vi "mian .vi"() -> ()   [LabVIEW 2013]
panel:
  out "机器ID":string="F3XS67WZ8BAQ"
  in  "密钥":u32=1308622971
  in  "VD":T1
  in  "PLC 系列":u8(ring) items=["1200.200.200SMART"=0, "S7-300"=2, "S7-400"=3]
  in  "PLC IP":string="192.168.3.200"
  in  "VW":T2={"VW0"=30, "VW2"=0, "VW4"=0, "VW6"=0, "VW8"=0, "VW10"=0, "VW12"=0, "VW14"=0, "VW16"=0, "VW18"=0, "VW20"=0, "VW22"=0, "VW24"=0, "VW26"=0, "VW28"=0, "VW30"=0, "VW32"=0, "VW34"=0, "VW36"=0, "VW38"=0, "VW40"=0, "VW42"=0, "VW44"=0, "VW46"=0}
  out "RMD":T3
  in  "WMD":T4
  out "RQD":T3={"Y20 2"=FALSE, "Y21 2"=FALSE, "Y22 2"=FALSE, "Y24 2"=FALSE, "Y23 2"=FALSE, "Y25 2"=FALSE, "Y26 2"=FALSE, "Y27 2"=FALSE, "Y10 2"=FALSE, "Y11 2"=FALSE, "Y12 2"=FALSE, "Y13 2"=FALSE, "Y14 2"=FALSE, "Y15 2"=FALSE, "Y16 2"=FALSE, "Y17 2"=FALSE, "Y0 2"=TRUE, "Y1 2"=TRUE, "Y2 2"=TRUE, "Y3 2"=TRUE, "Y4 2"=TRUE, "Y5 2"=FALSE, "Y6 2"=FALSE, "Y7 2"=FALSE, "Y30 2"=FALSE, "Y31 2"=FALSE, "Y32 2"=FALSE, "Y33 2"=FALSE, "Y34  2"=FALSE, "Y35  2"=FALSE, "Y36 2"=FALSE, "Y37 2"=FALSE}
  in  "WQD":T4
  out "RID":T5
  in  "停止":bool
  # "MX.0"
  # "QX.0-QX.7"
  # "IX.0-IX.7"
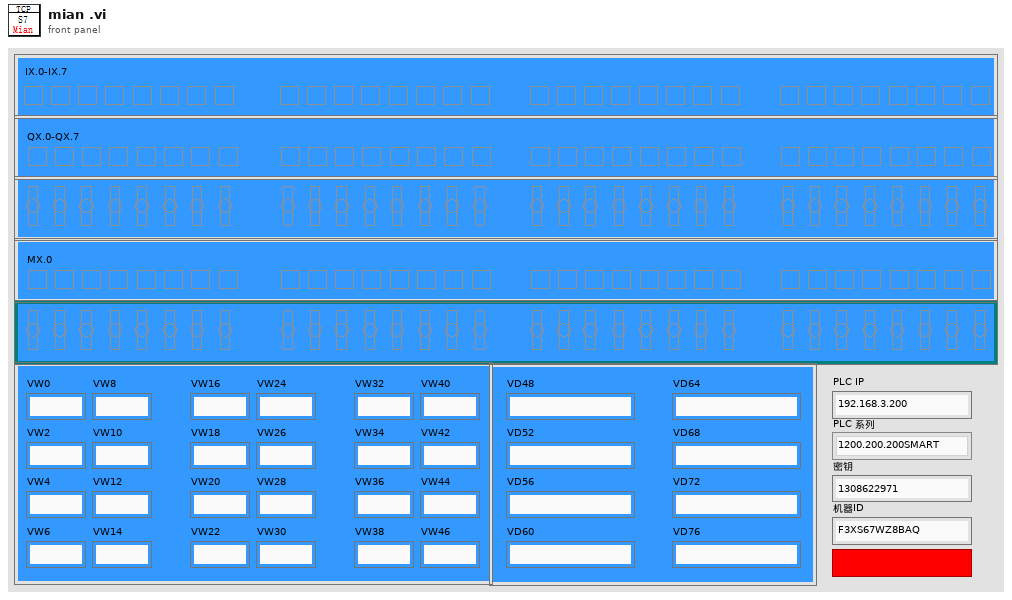
[diagram p1: front panel]
types:
  T1 = cluster{"VD48":u32, "VD52":u32, "VD56":u32, "VD60":u32, "VD64":u32, "VD68":u32, "VD72":u32, "VD76":u32}
  T2 = cluster{"VW0":u16, "VW2":u16, "VW4":u16, "VW6":u16, "VW8":u16, "VW10":u16, "VW12":u16, "VW14":u16, "VW16":u16, "VW18":u16, "VW20":u16, "VW22":u16, "VW24":u16, "VW26":u16, "VW28":u16, "VW30":u16, "VW32":u16, "VW34":u16, "VW36":u16, "VW38":u16, "VW40":u16, "VW42":u16, "VW44":u16, "VW46":u16}
  T3 = cluster{"Y20 2":bool, "Y21 2":bool, "Y22 2":bool, "Y24 2":bool, "Y23 2":bool, "Y25 2":bool, "Y26 2":bool, "Y27 2":bool, "Y10 2":bool, "Y11 2":bool, "Y12 2":bool, "Y13 2":bool, "Y14 2":bool, "Y15 2":bool, "Y16 2":bool, "Y17 2":bool, "Y0 2":bool, "Y1 2":bool, "Y2 2":bool, "Y3 2":bool, "Y4 2":bool, "Y5 2":bool, "Y6 2":bool, "Y7 2":bool, "Y30 2":bool, "Y31 2":bool, "Y32 2":bool, "Y33 2":bool, "Y34  2":bool, "Y35  2":bool, "Y36 2":bool, "Y37 2":bool}
  T4 = cluster{"Q3.0":bool, "Q3.1":bool, "Q3.2":bool, "Q3.3":bool, "Q3.4":bool, "Q3.5":bool, "Q3.6":bool, "Q3.7":bool, "Q2.0":bool, "Q2.1":bool, "Q2.2":bool, "Q2.3":bool, "Q2.4":bool, "Q2.5":bool, "Q2.6":bool, "Q2.7":bool, "Q1.0":bool, "Q1.1":bool, "Q1.2":bool, "Q1.3":bool, "Q1.4":bool, "Q1.5":bool, "Q1.6":bool, "Q1.7":bool, "Q0.0":bool, "Q0.1":bool, "Q0.2":bool, "Q0.3":bool, "Q0.4":bool, "Q0.5":bool, "Q0.6":bool, "Q0.7":bool}
  T5 = cluster{"X20":bool, "X21":bool, "X22":bool, "X24":bool, "X23":bool, "X25":bool, "X26":bool, "X27":bool, "X10":bool, "X11":bool, "X12":bool, "X13":bool, "X14":bool, "X15":bool, "X16":bool, " X17":bool, "X0":bool, "X1":bool, "X2":bool, "X3":bool, "X4":bool, "X5":bool, "X6":bool, "X7":bool, "X30":bool, "X31":bool, "X32":bool, "X33":bool, "X34 ":bool, "X35 ":bool, "X36":bool, "X37":bool}
  T6 = typedef "运行步骤控件.ctl" = enum16{"RI", "RQ", "RM", "RV"}
  T7 = cluster{"Boolean array[0]":bool, "Boolean array[1]":bool, "Boolean array[2]":bool, "Boolean array[3]":bool, "Boolean array[4]":bool, "Boolean array[5]":bool, "Boolean array[6]":bool, "Boolean array[7]":bool, "Boolean array[8]":bool, "Boolean array[9]":bool, "Boolean array[10]":bool, "Boolean array[11]":bool, "Boolean array[12]":bool, "Boolean array[13]":bool, "Boolean array[14]":bool, "Boolean array[15]":bool, "Boolean array[16]":bool, "Boolean array[17]":bool, "Boolean array[18]":bool, "Boolean array[19]":bool, "Boolean array[20]":bool, "Boolean array[21]":bool, "Boolean array[22]":bool, "Boolean array[23]":bool, "Boolean array[24]":bool, "Boolean array[25]":bool, "Boolean array[26]":bool, "Boolean array[27]":bool, "Boolean array[28]":bool, "Boolean array[29]":bool, "Boolean array[30]":bool, "Boolean array[31]":bool}
  T8 = cluster{"[0]":u32, "[1]":u32, "[2]":u32, "[3]":u32, "[4]":u32, "[5]":u32, "[6]":u32, "[7]":u32}
  T9 = cluster{"[0]":u16, "[1]":u16, "[2]":u16, "[3]":u16, "[4]":u16, "[5]":u16, "[6]":u16, "[7]":u16, "[8]":u16, "[9]":u16, "[10]":u16, "[11]":u16, "[12]":u16, "[13]":u16, "[14]":u16, "[15]":u16, "[16]":u16, "[17]":u16, "[18]":u16, "[19]":u16, "[20]":u16, "[21]":u16, "[22]":u16, "[23]":u16}
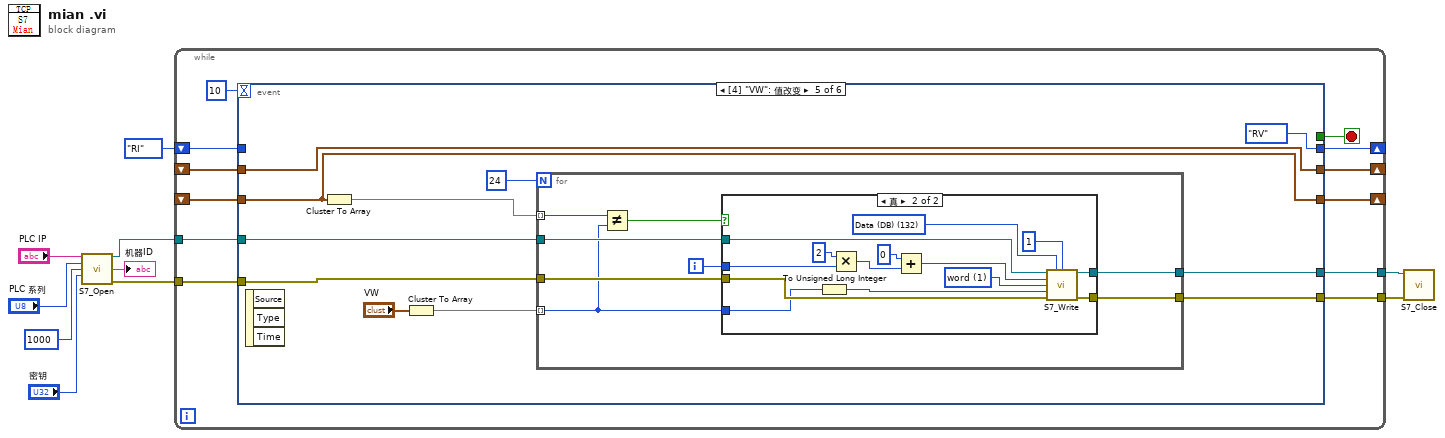
[diagram p0: block diagram]
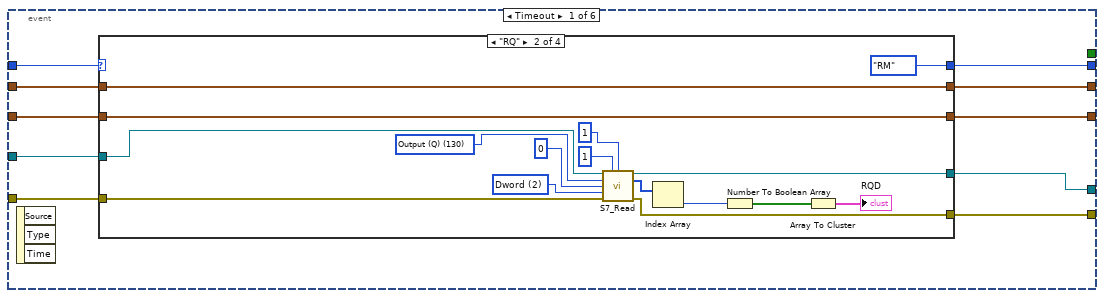
[diagram p2: hidden frame]
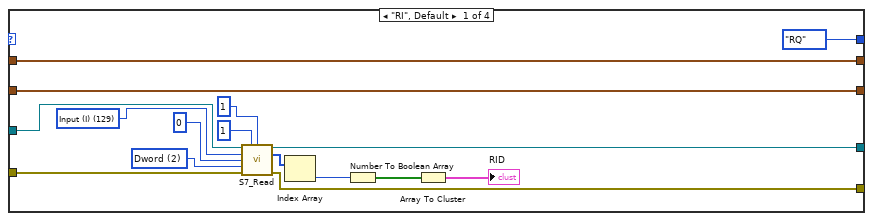
[diagram p3: hidden frame]
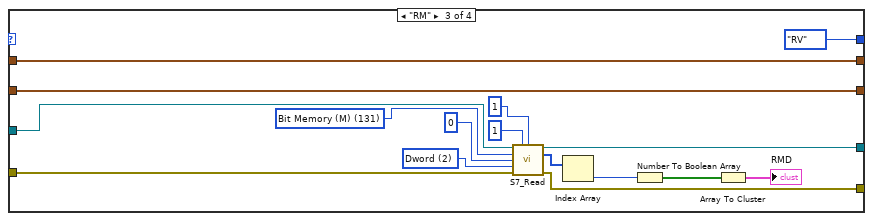
[diagram p4: hidden frame]
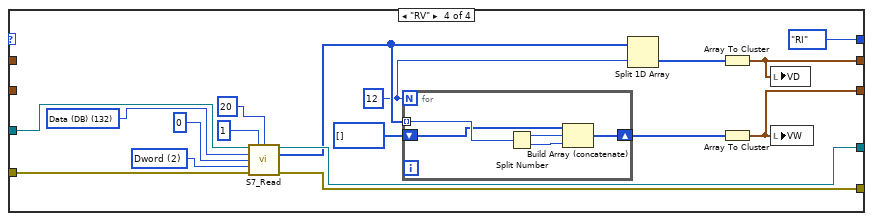
[diagram p5: hidden frame]
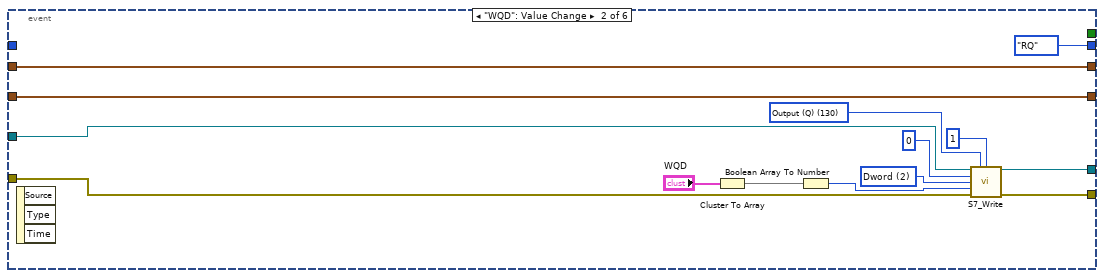
[diagram p6: hidden frame]
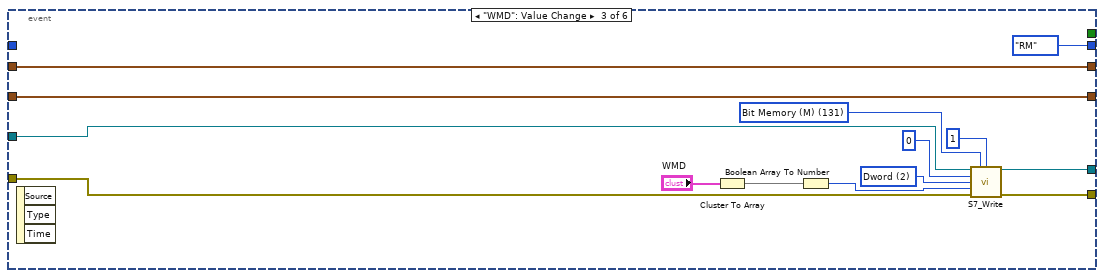
[diagram p7: hidden frame]
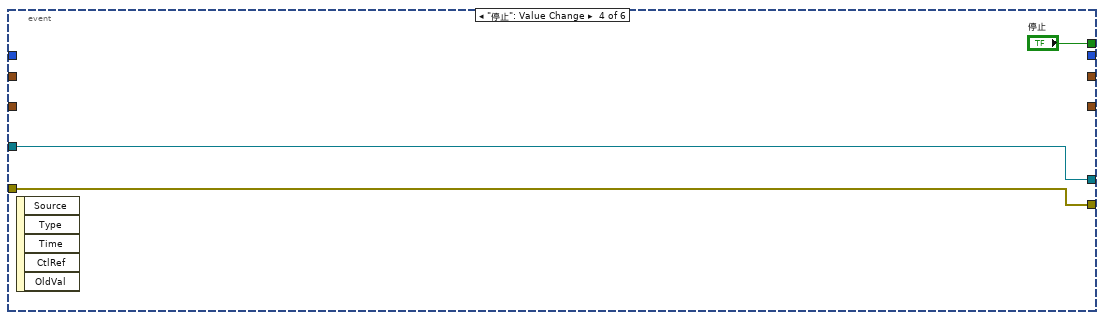
[diagram p8: hidden frame]
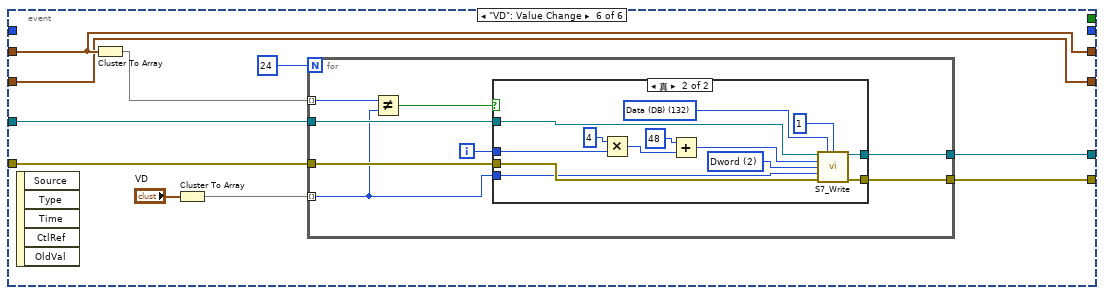
[diagram p10: hidden frame]
diagram:
  n1 = call "S7_Open.vi"("IP 地址"="PLC IP", "PLC 系列"="PLC 系列", "超时（MS）"=1000, "密钥"="密钥") -> ("TCP"=w9:refnum<k5>, "机器ID"=→"机器ID":string, "error out"=w8:errorcluster)  [unwired: 1 in, 8 out]
  n2 = while {
    tunnel: w9 -> [w21]
    tunnel: w8 -> [w20]
    tunnel: [w19] -> w7
    tunnel: [w18] -> w6
    shift-right: [w16] -> _
    shift-left: 运行步骤控件."RI" ("枚举") -> [w17]
    shift-right: [w15] -> _
    shift-left: _ -> [w13]
    shift-right: [w14] -> _
    shift-left: _ -> [w12]
    stop <- w11 stop-if-true
    n3 = event shown="[4] \"VW\": 值改变" {
      selector: _ -> [_ _ _ _ _ _]
      dyn-events: _ -> [_ _ _ _ _ _]
      timeout: 10 -> [_ _ _ _ _ _]
      tunnel: w21 -> [w32 w116 w122 w132 w142 w174]
      tunnel: w20 -> [w31 w115 w120 w131 w141 w173]
      tunnel: [w30 w114 w124 w132 w144 w172] -> w19
      tunnel: [w29 w113 w123 w131 w143 w171] -> w18
      tunnel: w17 -> [w28 _ _ _ _ _]
      tunnel: [w27 运行步骤控件."RQ" ("枚举") 运行步骤控件."RM" ("枚举") _ 运行步骤控件."RV" ("枚举") _] -> w16
      tunnel: [w26 w105 w119 _ w136 w169] -> w15
      tunnel: [w25 w104 w118 _ w135 w170] -> w14
      tunnel: w13 -> [w24 w105 w119 _ w136 w169]
      tunnel: w12 -> [w23 w104 w118 _ w135 w170]
      tunnel: [_ _ _ "停止" _ _] -> w11
      event Timeout {
        n4 = event-data() -> ()  [unwired: 4 out]
        n5 = case shown="\"RQ\"" w28 {
          tunnel: w32 -> [w44 w64 w72 w90]
          tunnel: w31 -> [w39 w63 w71 w89]
          tunnel: [w43 w62 w74 w92] -> w30
          tunnel: [w42 w61 w73 w91] -> w29
          tunnel: [运行步骤控件."RQ" ("枚举") 运行步骤控件."RM" ("枚举") 运行步骤控件."RV" ("枚举") 运行步骤控件."RI" ("枚举")] -> w27
          tunnel: [w34 w50 w66 w83] -> w26
          tunnel: [w33 w49 w65 w82] -> w25
          tunnel: w24 -> [w34 w50 w66 _]
          tunnel: w23 -> [w33 w49 w65 _]
          frame "RI", Default {
            w45 = u16 2 items=["byte", "word", "Dword"] ("数据类型")
            w41 = u8 129 items=["I/O (P)"=128, "Input (I)"=129, "Output (Q)"=130, "Bit Memory (M)"=131, "Data (DB)"=132, "Instance Data (DI)"=133, "Local Data (L)"=134, "Predecessor Local Data (VL)"=135] ("寄存器类型")
            n6 = call "S7_Read.vi"("TCP"=w44, "DB #"=u16 1, "读取长度"=u16 1, "寄存器类型"=w41, "起始地址"=u32 0, "数据类型"=w45, "error in"=w39) -> ("TCP"=w43:refnum<k5>, "数据"=w37:u32[], "error out"=w42:errorcluster)  [unwired: 6 out]
            n7 = Index Array(array=w37) -> (element=w36:u32)  [unwired: 1 in]
            n8 = Number To Boolean Array(number=w36) -> (Boolean array=w35:bool[])
            n9 = Array To Cluster(array=w35) -> (cluster=→"RID":T7)
          }
          frame "RQ" {
            w56 = u16 2 items=["byte", "word", "Dword"] ("数据类型")
            w58 = u8 130 items=["I/O (P)"=128, "Input (I)"=129, "Output (Q)"=130, "Bit Memory (M)"=131, "Data (DB)"=132, "Instance Data (DI)"=133, "Local Data (L)"=134, "Predecessor Local Data (VL)"=135] ("寄存器类型")
            n10 = call "S7_Read.vi"("TCP"=w64, "DB #"=u16 1, "读取长度"=u16 1, "寄存器类型"=w58, "起始地址"=u32 0, "数据类型"=w56, "error in"=w63) -> ("TCP"=w62:refnum<k5>, "数据"=w54:u32[], "error out"=w61:errorcluster)  [unwired: 6 out]
            n11 = Index Array(array=w54) -> (element=w53:u32)  [unwired: 1 in]
            n12 = Number To Boolean Array(number=w53) -> (Boolean array=w52:bool[])
            n13 = Array To Cluster(array=w52) -> (cluster=→"RQD":T7)
          }
          frame "RM" {
            w75 = u16 2 items=["byte", "word", "Dword"] ("数据类型")
            w79 = u8 131 items=["I/O (P)"=128, "Input (I)"=129, "Output (Q)"=130, "Bit Memory (M)"=131, "Data (DB)"=132, "Instance Data (DI)"=133, "Local Data (L)"=134, "Predecessor Local Data (VL)"=135] ("寄存器类型")
            n14 = call "S7_Read.vi"("TCP"=w72, "DB #"=u16 1, "读取长度"=u16 1, "寄存器类型"=w79, "起始地址"=u32 0, "数据类型"=w75, "error in"=w71) -> ("TCP"=w74:refnum<k5>, "数据"=w68:u32[], "error out"=w73:errorcluster)  [unwired: 6 out]
            n15 = Index Array(array=w68) -> (element=w70:u32)  [unwired: 1 in]
            n16 = Number To Boolean Array(number=w70) -> (Boolean array=w69:bool[])
            n17 = Array To Cluster(array=w69) -> (cluster=→"RMD":T7)
          }
          frame "RV" {
            w93 = u16 2 items=["byte", "word", "Dword"] ("数据类型")
            w97 = u8 132 items=["I/O (P)"=128, "Input (I)"=129, "Output (Q)"=130, "Bit Memory (M)"=131, "Data (DB)"=132, "Instance Data (DI)"=133, "Local Data (L)"=134, "Predecessor Local Data (VL)"=135] ("寄存器类型")
            w81 = 12
            n18 = call "S7_Read.vi"("TCP"=w90, "DB #"=u16 1, "读取长度"=u16 20, "寄存器类型"=w97, "起始地址"=u32 0, "数据类型"=w93, "error in"=w89) -> ("TCP"=w92:refnum<k5>, "数据"=w86:u32[], "error out"=w91:errorcluster)  [unwired: 6 out]
            n19 = for {
              N: w81 -> [_]
              tunnel: w86 -> [w102] mode=indexing
              shift-right: [w101] -> w85
              shift-left: u16[] [] -> [w100]
              n20 = Split Number(x=w102) -> (hi(x)=w99:u16, lo(x)=w98:u16)
              n21 = Build Array (concatenate)(w100, w99, w98) -> (w101:u16[])
            }
            n22 = Split 1D Array(array=w86, index=w81) -> (second subarray=w84:u32[])  [unwired: 1 out]
            n23 = Array To Cluster(array=w84) -> (cluster=w82:T8)
            n24 = Array To Cluster(array=w85) -> (cluster=w83:T9)
            n25 = local write "VD"(w82) -> ()
            n26 = local write "VW"(w83) -> ()
          }
        }
      }
      event "WQD": Value Change {
        w109 = u16 2 items=["byte", "word", "Dword"] ("数据类型")
        w112 = u8 130 items=["I/O (P)"=128, "Input (I)"=129, "Output (Q)"=130, "Bit Memory (M)"=131, "Data (DB)"=132, "Instance Data (DI)"=133, "Local Data (L)"=134, "Predecessor Local Data (VL)"=135] ("寄存器类型")
        n27 = event-data() -> ()  [unwired: 4 out]
        n28 = Cluster To Array(cluster="WQD") -> (array=w107:bool[])
        n29 = Boolean Array To Number(Boolean array=w107) -> (number=w106:u32)
        n30 = call "S7_Write.vi"("TCP"=w116, "寄存器类型"=w112, "DB #"=u16 1, "写入地址"=u32 0, "数据类型"=w109, "写入数据"=w106, "error in"=w115) -> ("TCP"=w114:refnum<k5>, "error out"=w113:errorcluster)  [unwired: 7 out]
      }
      event "WMD": Value Change {
        w127 = u16 2 items=["byte", "word", "Dword"] ("数据类型")
        w130 = u8 131 items=["I/O (P)"=128, "Input (I)"=129, "Output (Q)"=130, "Bit Memory (M)"=131, "Data (DB)"=132, "Instance Data (DI)"=133, "Local Data (L)"=134, "Predecessor Local Data (VL)"=135] ("寄存器类型")
        n31 = event-data() -> ()  [unwired: 4 out]
        n32 = Cluster To Array(cluster="WMD") -> (array=w126:bool[])
        n33 = Boolean Array To Number(Boolean array=w126) -> (number=w125:u32)
        n34 = call "S7_Write.vi"("TCP"=w122, "寄存器类型"=w130, "DB #"=u16 1, "写入地址"=u32 0, "数据类型"=w127, "写入数据"=w125, "error in"=w120) -> ("TCP"=w124:refnum<k5>, "error out"=w123:errorcluster)  [unwired: 7 out]
      }
      event "停止": Value Change {
        n35 = event-data() -> ()  [unwired: 6 out]
      }
      event "VW": Value Change {
        n36 = event-data() -> ()  [unwired: 4 out]
        n37 = Cluster To Array(cluster=w136) -> (array=w138:u16[])
        n38 = Cluster To Array(cluster="VW") -> (array=w137:u16[])
        n39 = for {
          N: 24 -> [_]
          tunnel: [w152] -> w144
          tunnel: [w151] -> w143
          tunnel: w142 -> [w150]
          tunnel: w141 -> [w149]
          tunnel: w138 -> [w148] mode=indexing
          tunnel: w137 -> [w146] mode=indexing
          i -> [w145]
          n40 = Not Equal?(x=w148, y=w146) -> (x != y?=w147:bool)
          n41 = case shown="真" w147 {
            tunnel: [w154 w165] -> w152
            tunnel: [w153 w164] -> w151
            tunnel: w150 -> [w154 w163]
            tunnel: w149 -> [w153 w162]
            tunnel: w146 -> [_ w157]
            tunnel: w145 -> [_ w159]
            frame False {
            }
            frame True {
              w166 = u16 1 items=["byte", "word", "Dword"] ("数据类型")
              w168 = u8 132 items=["I/O (P)"=128, "Input (I)"=129, "Output (Q)"=130, "Bit Memory (M)"=131, "Data (DB)"=132, "Instance Data (DI)"=133, "Local Data (L)"=134, "Predecessor Local Data (VL)"=135] ("寄存器类型")
              n42 = To Unsigned Long Integer(number=w157) -> (unsigned 32bit integer=w156:u32)
              n43 = Multiply(x=u32 2, y=w159) -> (x*y=w160:u32)
              n44 = Add(x=u32 0 ("写入地址"), y=w160) -> (x+y=w155:u32)
              n45 = call "S7_Write.vi"("TCP"=w163, "寄存器类型"=w168, "DB #"=u16 1, "写入地址"=w155, "数据类型"=w166, "写入数据"=w156, "error in"=w162) -> ("TCP"=w165:refnum<k5>, "error out"=w164:errorcluster)  [unwired: 7 out]
            }
          }
        }
      }
      event "VD": Value Change {
        n46 = event-data() -> ()  [unwired: 6 out]
        n47 = Cluster To Array(cluster=w170) -> (array=w177:u32[])
        n48 = Cluster To Array(cluster="VD") -> (array=w176:u32[])
        n49 = for {
          N: 24 -> [_]
          tunnel: [w186] -> w172
          tunnel: [w185] -> w171
          tunnel: w174 -> [w184]
          tunnel: w173 -> [w183]
          tunnel: w177 -> [w182] mode=indexing
          tunnel: w176 -> [w180] mode=indexing
          i -> [w179]
          n50 = Not Equal?(x=w182, y=w180) -> (x != y?=w181:bool)
          n51 = case shown="真" w181 {
            tunnel: [w188 w198] -> w186
            tunnel: [w187 w197] -> w185
            tunnel: w184 -> [w188 w196]
            tunnel: w183 -> [w187 w195]
            tunnel: w180 -> [_ w189]
            tunnel: w179 -> [_ w192]
            frame False {
            }
            frame True {
              w199 = u16 2 items=["byte", "word", "Dword"] ("数据类型")
              w201 = u8 132 items=["I/O (P)"=128, "Input (I)"=129, "Output (Q)"=130, "Bit Memory (M)"=131, "Data (DB)"=132, "Instance Data (DI)"=133, "Local Data (L)"=134, "Predecessor Local Data (VL)"=135] ("寄存器类型")
              n52 = Multiply(x=u32 4, y=w192) -> (x*y=w193:u32)
              n53 = Add(x=u32 48 ("写入地址"), y=w193) -> (x+y=w190:u32)
              n54 = call "S7_Write.vi"("TCP"=w196, "寄存器类型"=w201, "DB #"=u16 1, "写入地址"=w190, "数据类型"=w199, "写入数据"=w189, "error in"=w195) -> ("TCP"=w198:refnum<k5>, "error out"=w197:errorcluster)  [unwired: 7 out]
            }
          }
        }
      }
    }
  }
  n55 = call "S7_Close.vi"("error in"=w6, "TCP Connection Ref"=w7) -> ()  [unwired: 10 out]
